vi "stopCalibrationPopUp.vi"() -> ()   [LabVIEW 2013, in "main.lvlib"]
uses:
  main.lvlib
  Controls/Enum User Events.ctl
panel:
  in  "System Stop Button":bool
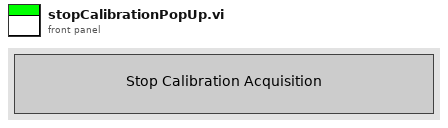
[diagram p1: front panel]
types:
  T1 = typedef "main.lvlib/Enum User Events.ctl" = enum16{"User Event", "Init"}
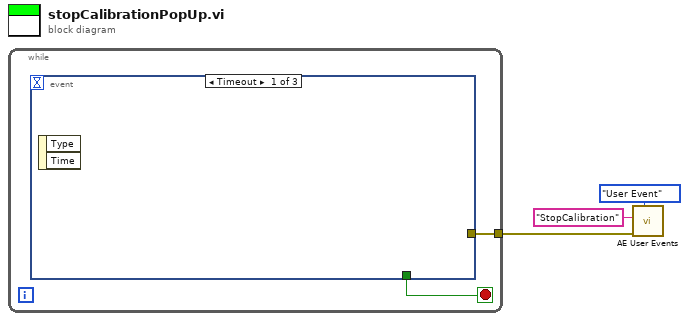
[diagram p0: block diagram]
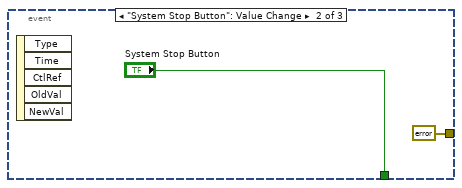
[diagram p2: hidden frame]
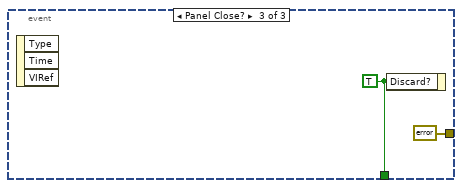
[diagram p3: hidden frame]
diagram:
  n1 = while {
    tunnel: [w4] -> w1
    stop <- w5 stop-if-true
    n2 = event shown="[0] Timeout" {
      selector: _ -> [_ _ _]
      dyn-events: _ -> [_ _ _]
      timeout: _ -> [_ _ _]
      tunnel: [_ "System Stop Button" w9] -> w5
      tunnel: [_ errorcluster {"status"=FALSE, "code"=0, "source"=""} ("error in (no error)") errorcluster {"status"=FALSE, "code"=0, "source"=""} ("error in (no error)")] -> w4
      event Timeout {
        n3 = event-data() -> ()  [unwired: 1 in, 2 out]
      }
      event "System Stop Button": Value Change {
        n4 = event-data() -> ()  [unwired: 1 in, 5 out]
      }
      event Panel Close? {
        w9 = TRUE ("Discard?")
        n5 = event-data() -> ()  [unwired: 1 in, 3 out]
        n6 = event-data("Discard?"=w9) -> ()  [unwired: 1 in, 1 out]
      }
    }
  }
  n7 = call "AE User Events.vi"("Action"=Enum_User_Events."User Event", "error in (no error)"=w1, "User Event"="StopCalibration") -> ()  [unwired: 7 in, 2 out]
